vi "Create Frame Pattern Script.vi"(8 "error in (no error)":errorcluster, 9 "ChipID":u8, 10 "Frame_Data":T1={"Pattern_Name"="", "Operation Mode"=enum."Normal", "BurstLength"=enum."0", "FSN"=0, "Start_Addr"=0, "Data"=[], "R/W?"=enum."Read", "Opcode"=[], "ChipID"=1, "num of wait cycle of read"=0} {"Data" format="%x"; "Start_Addr" format="%x"}, 11 "BML_Frame_Data in":refnum<class "BML_Frame_Data.lvclass">) -> (0 "error out":errorcluster, 3 "BML_Frame_Data out":refnum<class "BML_Frame_Data.lvclass">)   [LabVIEW 2018, in "BML_Frame_Data.lvclass"]
uses:
  BML_Frame_Data.lvclass
  C:/P4 Workspace/PC Client/Solutions/5g_eap/HiSi/trunk/1.0/BML_Pattern_Gen_Refactor/Classes/BML_Frame_Root/BML_Frame_Root.lvclass
  Config_Read/Frame_Data.ctl
  Config_Read/OperationMode.ctl
  Config_Read/BurstLength.ctl
  Config_Read/RW_Option.ctl
  BML_Frame_Root/BML_Frame_Root.lvclass/BML_Frame_Root.ctl
  BML_Frame_Root/BML_Frame_Root.lvclass
  Config_Read/Config_Read_BML.lvclass
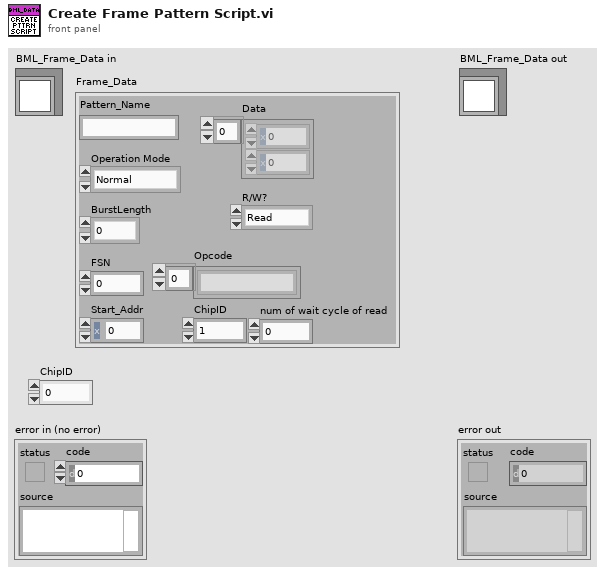
[diagram p1: front panel]
types:
  T1 = typedef "Config_Read_BML.lvclass/Frame_Data.ctl" = cluster{"Pattern_Name":string, "Operation Mode":T2, "BurstLength":T3, "FSN":u8, "Start_Addr":u16, "Data":u8[], "R/W?":T4, "Opcode":string[], "ChipID":u8, "num of wait cycle of read":i8}
  T2 = typedef "Config_Read_BML.lvclass/OperationMode.ctl" = enum8{"Normal", "ImmeEffect", "InitSlaveID", "LoadData"}
  T3 = typedef "Config_Read_BML.lvclass/BurstLength.ctl" = enum8{"0", "2", "3", "4", "5", "8", "16", "32"}
  T4 = typedef "Config_Read_BML.lvclass/RW_Option.ctl" = enum16{"Read", "Write", "R/W"}
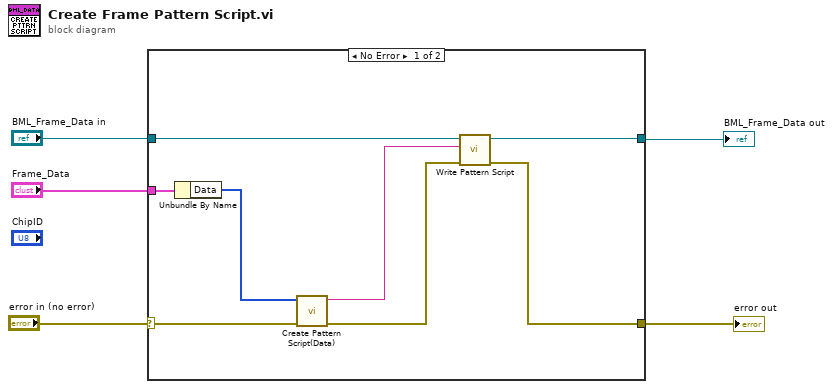
[diagram p0: block diagram]
diagram:
  n1 = case shown="No Error" "error in (no error)" {
    selector: "error in (no error)" -> [w7 w15]
    tunnel: "BML_Frame_Data in" -> [w12 w14]
    tunnel: [w10 w15] -> w2
    tunnel: [w11 w14] -> w4
    tunnel: "Frame_Data" -> [w13 _]
    frame No Error {
      n2 = Unbundle By Name(w13) -> ("Data"=w9:u8[])
      n3 = call "Create Pattern Script(Data).vi"("error in (no error)"=w7, "Data"=w9) -> ("error out"=w6:errorcluster, "String"=w8:string)  [unwired: 8 in]
      n4 = call "Write Pattern Script.vi"("error in (no error)"=w6, "Pattern Script"=w8, "BML_Frame_Root in"=w12) -> ("error out"=w10:errorcluster, "BML_Frame_Root out"=w11:refnum<class "BML_Frame_Data.lvclass">)  [unwired: 7 in]
    }
    frame Error {
    }
  }
  "error out" <- w2
  "BML_Frame_Data out" <- w4
